vi "set_duty.vi"(8 "error in (no error)":errorcluster, 10 "Value":dbl, 11 "VISA Refnum in":refnum<visa-resource-name>) -> (0 "error out":errorcluster, 3 "VISA Refnum out":refnum<visa-resource-name>)   [LabVIEW 2015]
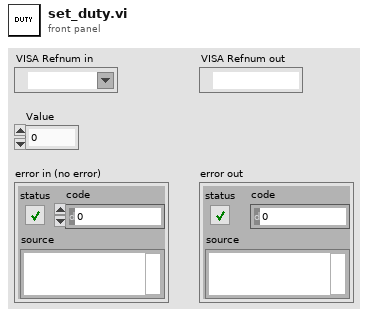
[diagram p1: front panel]
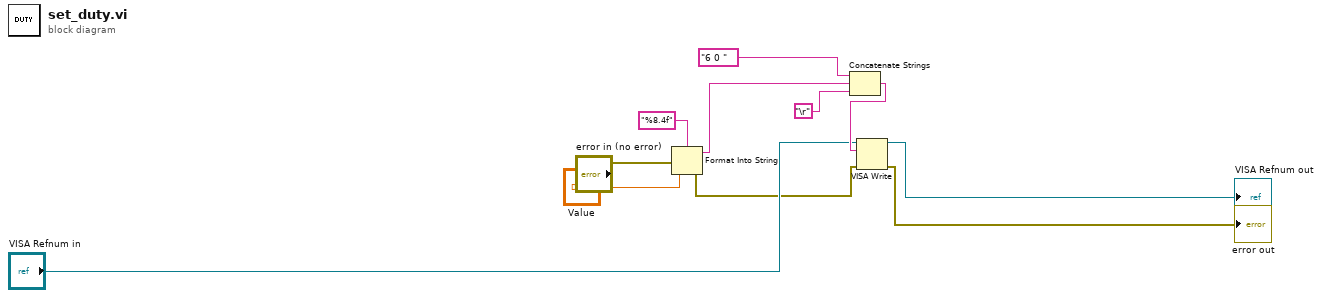
[diagram p0: block diagram]
diagram:
  n1 = Format Into String(format string="%8.4f", error in="error in (no error)", "Value") -> (resulting string=w10:string, error out=w2:errorcluster)  [unwired: 1 in]
  n2 = Concatenate Strings("6 0 " ("string"), w10, "\r") -> (w11:string)
  n3 = VISA Write(VISA resource name="VISA Refnum in", write buffer=w11, error in (no error)=w2) -> (VISA resource name out=→"VISA Refnum out":refnum<visa-resource-name>, error out=→"error out":errorcluster)  [unwired: 1 out]
